vi "SubRoutine Stepper.vi"(0 "Current Step in":i32, 5 "# of Steps":i32, 7 "Cycles Completed in":u32, 9 "Cycles Required":u32) -> (4 "Current Step out":i32, 8 "Cycles Completed out":u32, 15 "Run Run Step":bool)   [LabVIEW 2013]
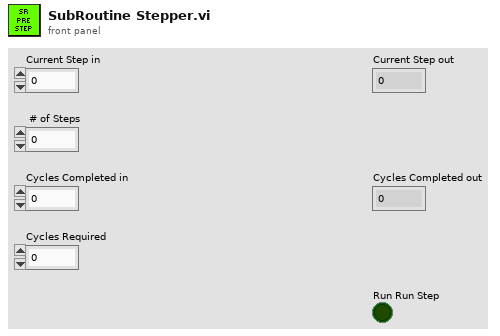
[diagram p1: front panel]
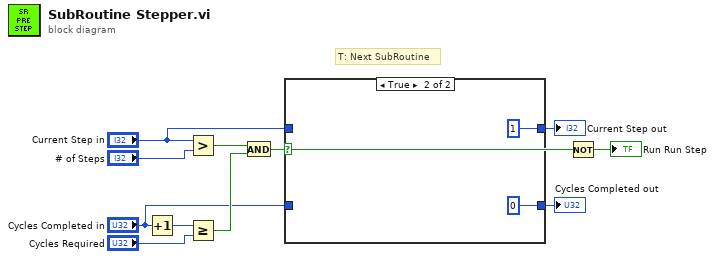
[diagram p0: block diagram]
diagram:
  # "T: Next SubRoutine"
  n1 = Increment(x="Cycles Completed in") -> (x+1=w10:u32)
  n2 = Greater?(x="Current Step in", y="# of Steps") -> (0:w8:bool)
  n3 = Greater Or Equal?(x=w10, y="Cycles Required") -> (x >= y?=w7:bool)
  n4 = And(x=w8, y=w7) -> (x .and. y?=w5:bool)
  n5 = case shown="True" w5 {
    tunnel: "Current Step in" -> [w13 _]
    tunnel: [w13 1 ("Current Step in")] -> w3
    tunnel: [w12 u32 0 ("Cycles Completed in")] -> w1
    tunnel: "Cycles Completed in" -> [w12 _]
    frame False {
    }
    frame True {
    }
  }
  "Current Step out" <- w3
  "Cycles Completed out" <- w1
  n6 = Not(x=w5) -> (.not. x?=→"Run Run Step":bool)
